vi "PDF Standard Kopf IAGnG.vi"(4 "Zeitstempel":timestamp, 5 "Gaschflasche Cluster":T2, 6 "Oprtionen Cluster":T5, 7 "Gas Komponente":cluster{"Komponente:":T4, "Konzentration":dbl} {"Konzentration" format="%#.6f"}, 8 "error in (no error)":errorcluster caption="Fehler (Eingang, kein Fehler)", 9 "LIN Pototokoll-Cluster (opotional)":T6 {"zusätzliche Zeitdauer Erster Punkt" format="%#_5g"; "Lin Modus" items=["Cal Gas to PNS", "Cal Gas to Samplepoint", "Measure"]; "Gas Ablaufdatum" format="%<%d.%m.%Y>T"; "HovaCAL Flow AutoLin"."HovaCAL Flow Input Cluster" format="%.2f"; "Gasflasche" items=["----"=10000, "IAG MG"=0, "IAG NH3 3000"=1, "IAG NH3 2000"=2, "IAG NH3 200"=3]; "Conditions:" items=["field", "laboratory"]; "Kalibrierauswahl" items=["Inaktiv", "Aktiv"]; "Anzahl Stufen" format="%#_5g"; "Zeitdauer Stufe" format="%#_5g"; "Verdünnungsgas" items=["N2", "O2"]; "Komponentenauswahl"."Konzentration" format="%#.6f"; "Gasnummer:" min=1 max=5; "Prüfgas Konzentration" format="%#.6f"; "Polynomkoeff." format="%#_18f"}, 10 "Analysator":string, 11 "Bearbeiter/in":string) -> (0 "error out":errorcluster caption="Fehler (Ausgang)", 1 "Size Cluster":T1={"Header Size"=0, "Column Ratio left"=[40.0, 60.0]}, 2 "Header Values":T3[](array[typedef]), 3 "Header Labels":string[](array[string]))   [LabVIEW 2020, in "Linearisierung v2.lvlib" / "Protokoll.lvlib"]
uses:
  Protokoll.lvlib
  Lin-Polynom Daten.ctl
  KomponentenArray.ctl
  Visualisierungs Elemente/Auswahlfeld.ctl
  Visualisierungs Elemente/Zahlen-Eingabefeld.ctl
  EPA Optionsfeld.ctl
  Gasteiler/HovaCal/AutoLin Hovacal.ctl
  Kalibrieroption.ctl
  EPA1065-307/Condition.ctl
  Seiten/System Einstellungen V2/Konfig Gasflasche.ctl
  Seiten/System Einstellungen V2/Gasflasche Auswahl.ctl
  Gasteiler/HovaCAL_Interface/Controls/Flow Einstellung.ctl
  Gasteiler/HovaCAL_Interface/Controls/Pump state.ctl
  Seiten/CalGas Aufschaltung/Lin Modus.ctl
  PDF_Interface/PDF Protokoll Standard Kopf Optionen.ctl
  Visualisierungs Elemente/String - Ausgabefeld.ctl
  PDF_Interface/PDF Protokoll Standard Kopf Gasflasche Auswahl.ctl
  Gasteiler/Aktionen FGV Gasteiler Daten.ctl
  Seiten/FT-IR/FGV FT-IR Gasliste Aktionen.ctl
  Seiten/FT-IR/FGV FT-IR Aktionen.ctl
  Gasteiler/Gasteiler.lvlib
  Seiten/FT-IR/FT-IR.lvlib
  PDF_Interface/PDF Interface.lvlib
  Linearisierung v2.lvlib
  Gasteiler/HovaCal/HovaCal.lvlib
  EPA1065-307/Linearity verification 1065-307.lvlib
  Seiten/System Einstellungen V2/System Einstellungen V2.lvlib
  Gasteiler/HovaCAL_Interface/Controls/Controls.lvlib
  Seiten/CalGas Aufschaltung/CalGas Aufschaltung.lvlib
panel:
  # "%"
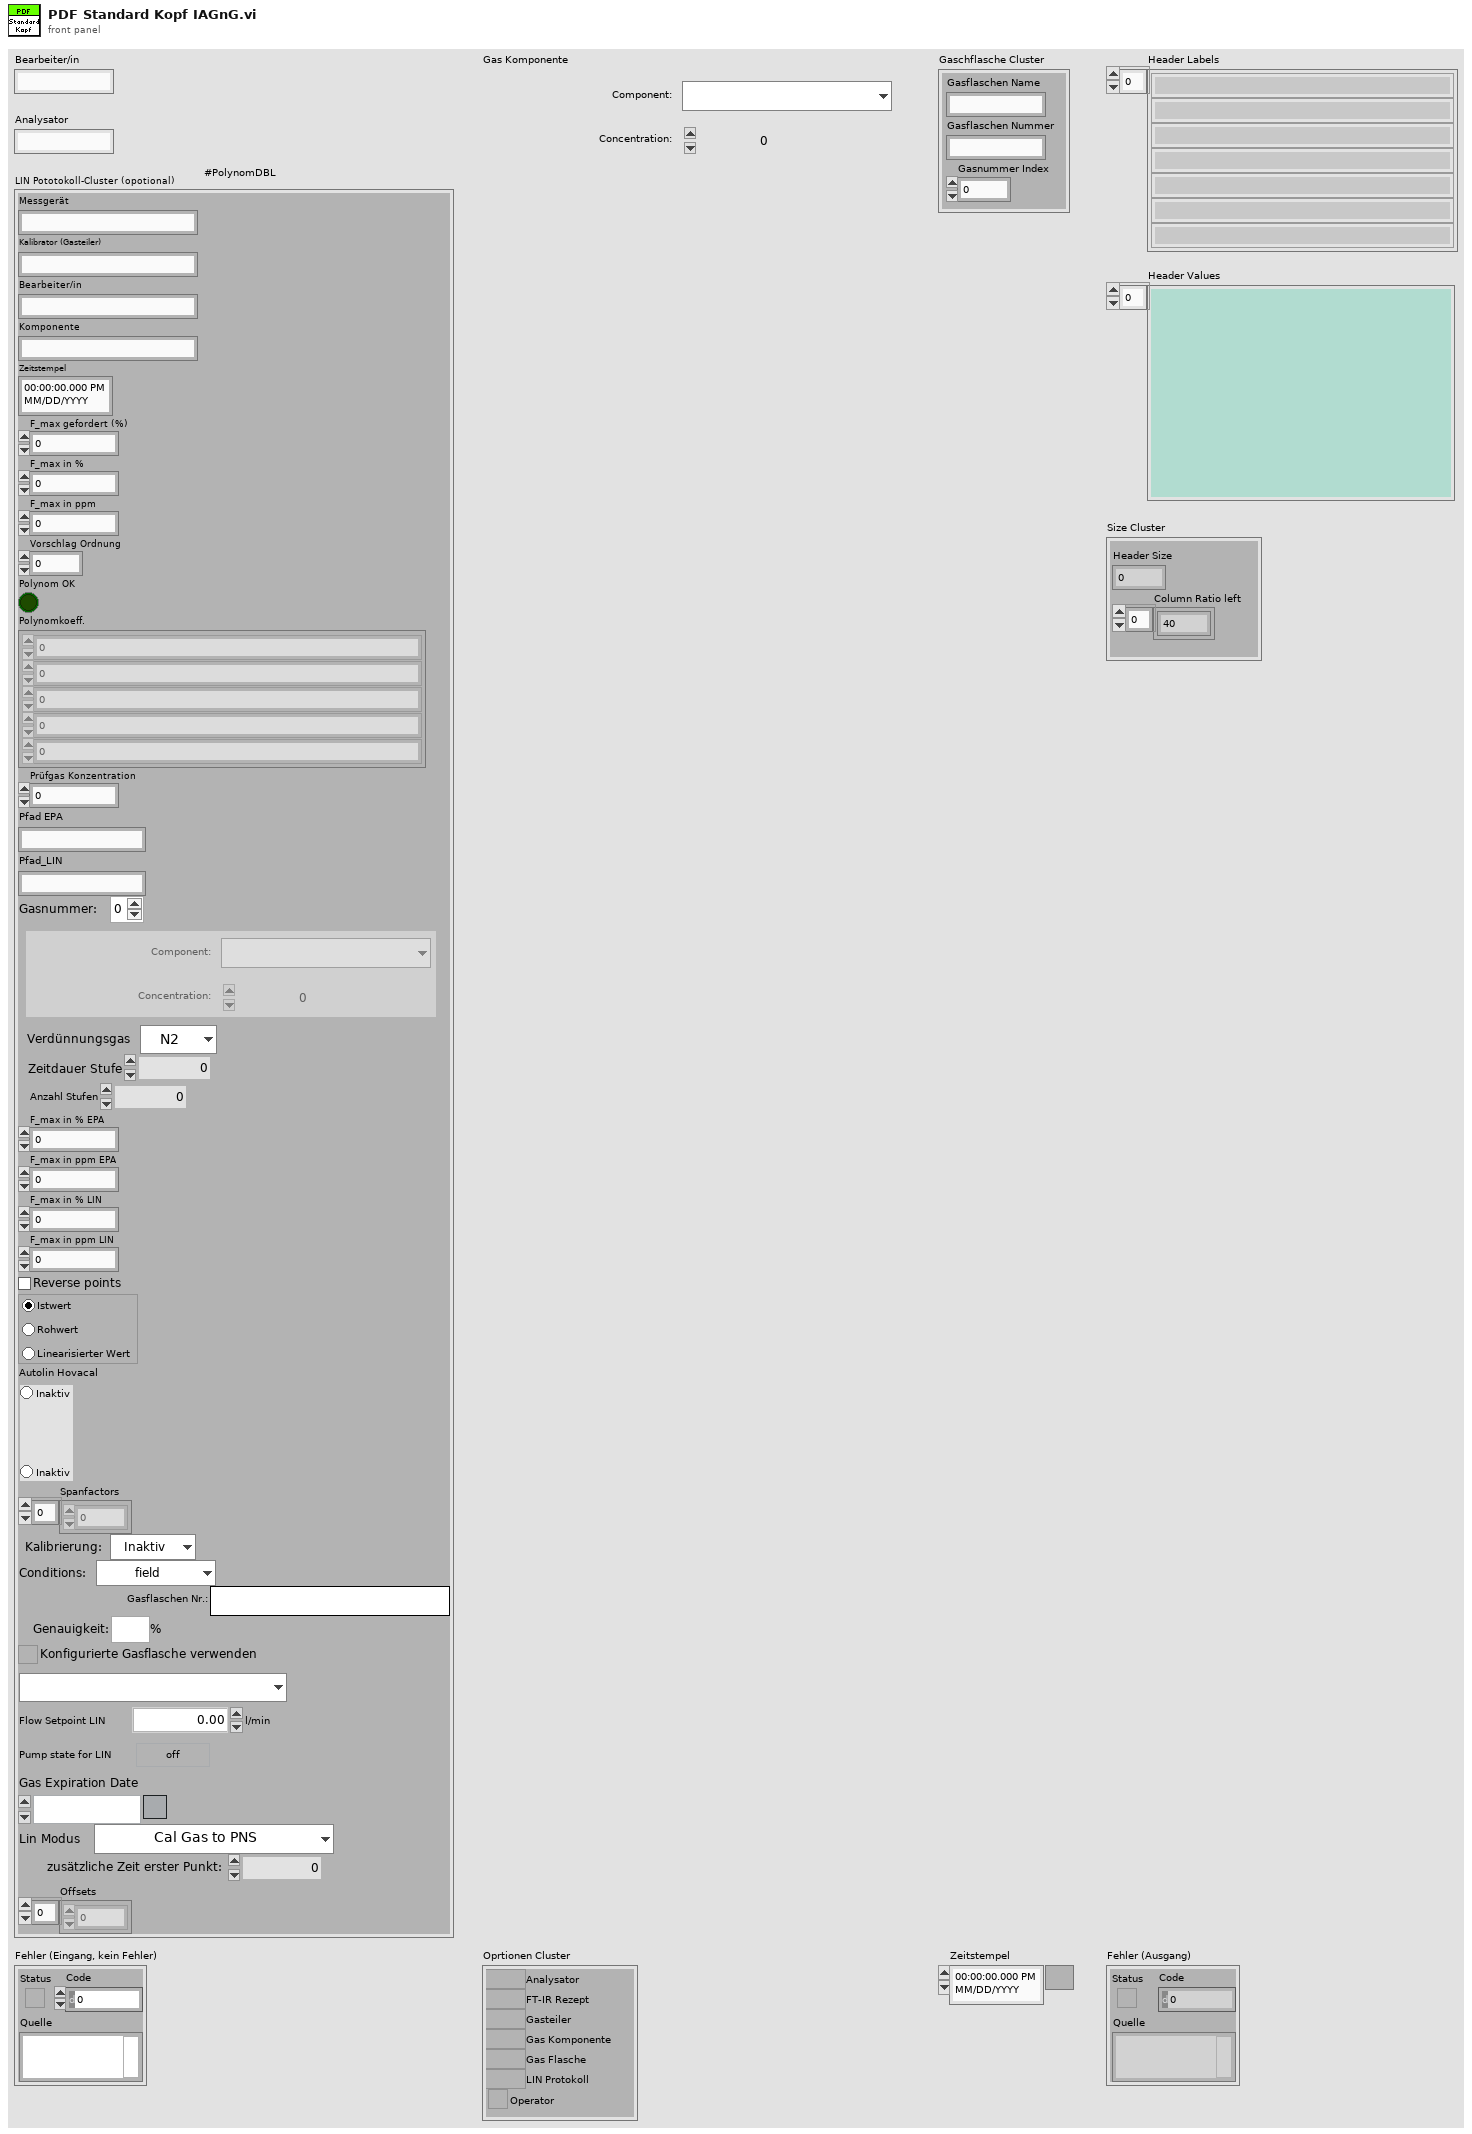
[diagram p1: front panel]
types:
  T1 = cluster{"Header Size":i32, "Column Ratio left":sgl[]}
  T2 = typedef "PDF Interface.lvlib/PDF Protokoll Standard Kopf Gasflasche Auswahl.ctl" = cluster{"Gasflaschen Name":string, "Gasflaschen Nummer":string, "Gasnummer Index":i32}
  T3 = typedef "String - Ausgabefeld.ctl" = string
  T4 = typedef "Auswahlfeld.ctl" = u16
  T5 = typedef "PDF Interface.lvlib/PDF Protokoll Standard Kopf Optionen.ctl" = cluster{"Analysator":bool, "FT-IR Rezept":bool, "Gasteiler":bool, "Gas Komponente":bool, "Gas Flasche":bool, "LIN Protokoll":bool, "Operator":bool}
  T6 = typedef "Linearisierung v2.lvlib/Lin-Polynom Daten.ctl" = cluster{"Messgerät":string, "Kalibrator (Gasteiler)":string, "Bearbeiter/in":string, "Komponente":string, "Zeitstempel":timestamp, "F_max gefordert (%)":sgl, "F_max in %":sgl, "F_max in ppm":sgl, "Vorschlag Ordnung":i32, "Polynom OK":bool, "Polynomkoeff.":dbl[], "Prüfgas Konzentration":dbl, "Pfad EPA":string, "Pfad_LIN":string, "Gasnummer:":u8, "Komponentenauswahl":T7, "Verdünnungsgas":T8, "Zeitdauer Stufe":T9, "Anzahl Stufen":T9, "F_max in % EPA":sgl, "F_max in ppm EPA":sgl, "F_max in % LIN":sgl, "F_max in ppm LIN":sgl, "Punkte umkehren":bool, "EPA Optionsfeld":T10, "Autolin Hovacal":T11, "Spanfactors":sgl[], "Kalibrierauswahl":T12, "Conditions:":T13, "Gasflaschen Nr.:":string, "Bottle Accuracy":dbl, "Konfig Gasflasche":T14, "Gasflasche":T15, "HovaCAL Flow AutoLin":T16, "MFC Output":T17, "Gas Ablaufdatum":timestamp, "Lin Modus":T18, "zusätzliche Zeitdauer Erster Punkt":sgl, "Offsets":sgl[]}
  T7 = typedef "Linearisierung v2.lvlib/KomponentenArray.ctl" = cluster{"Komponente:":T4, "Konzentration":dbl}[]
  T8 = typedef "Linearisierung v2.lvlib/Gasteiler.lvlib/Prüfgas in.ctl" = u16
  T9 = typedef "Zahlen-Eingabefeld.ctl" = sgl
  T10 = typedef "Linearisierung v2.lvlib/EPA Optionsfeld.ctl" = enum32{"Istwert", "Rohwert", "Linearisierter Wert"}
  T11 = typedef "Linearisierung v2.lvlib/Gasteiler.lvlib/HovaCal.lvlib/AutoLin Hovacal.ctl" = enum32{"Keine Auswahl", "Optionsauswahl 1", "Optionsauswahl 2"}
  T12 = typedef "Linearisierung v2.lvlib/Kalibrieroption.ctl" = u16
  T13 = typedef "Linearisierung v2.lvlib/Linearity verification 1065-307.lvlib/Condition.ctl" = u16
  T14 = typedef "System Einstellungen V2.lvlib/Konfig Gasflasche.ctl" = bool
  T15 = typedef "System Einstellungen V2.lvlib/Gasflasche Auswahl.ctl" = u16
  T16 = typedef "Linearisierung v2.lvlib/Gasteiler.lvlib/HovaCAL_Interface.lvlib/Controls.lvlib/Flow Einstellung.ctl" = cluster{"HovaCAL Flow Input Cluster":dbl}
  T17 = typedef "Linearisierung v2.lvlib/Gasteiler.lvlib/HovaCAL_Interface.lvlib/Controls.lvlib/Pump state.ctl" = cluster{"Run":bool}
  T18 = typedef "CalGas Aufschaltung.lvlib/Lin Modus.ctl" = u16
  T19 = typedef "FT-IR.lvlib/FGV FT-IR Aktionen.ctl" = enum16{"lesen", "NOG setzen", "NOS setzen", "Initialisieren", "speichern", "ALLES setzen", "FT-IR Spektrum loggen", "Komm Stoppen", "Spektrum LogKonfig"}
  T20 = typedef "FT-IR.lvlib/FGV FT-IR Gasliste Aktionen.ctl" = enum16{"lesen", "Gasliste FT-IR", "Gasliste ausgelesen", "laden", "speichern", "löschen"}
  T21 = typedef "Linearisierung v2.lvlib/Gasteiler.lvlib/Aktionen FGV Gasteiler Daten.ctl" = enum16{"lesen", "Gasteiler Daten", "Seriellen Param.", "MB-Endwert", "laden", "speichern", "Anforderung", "TCP", "Aufzeichnung Start"}
  T22 = typedef "Linearisierung v2.lvlib/Gasteiler.lvlib/Gasteiler Daten.ctl" = cluster{"Gasteiler":T23, "Gasteiler Stufen":T24, "Gasteiler Type":T25, "Konfig Gasteiler":T26, "Gasteiler Span Eingänge":u16}
  T23 = typedef "String - Eingabefeld.ctl" = string
  T24 = typedef "Linearisierung v2.lvlib/Gasteiler.lvlib/Gasteiler Stufen.ctl" = u16
  T25 = typedef "Linearisierung v2.lvlib/GasteilerType.ctl" = u16
  T26 = typedef "System Einstellungen V2.lvlib/Gasteiler Auswahl.ctl" = u16
  T27 = cluster{"Zeitstempel":timestamp, "Current Recipe":string, "Konfig Gasteiler":T26, "Aktuelle Gasliste gesamt":T3[]}
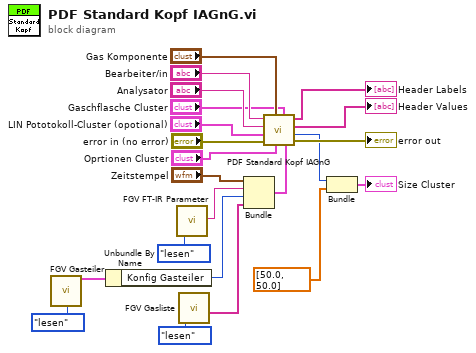
[diagram p0: block diagram]
diagram:
  n1 = call "FGV Gasteiler.vi"("Aktionen"=Aktionen_FGV_Gasteiler_Daten."lesen") -> ("Gasteiler Daten"=w21:T22)  [unwired: 11 in, 7 out]
  n2 = Unbundle By Name(w21) -> ("Konfig Gasteiler"=w14:T26)
  n3 = call "FGV FT-IR Parameter.vi"("Aktion"=FGV_FT-IR_Aktionen."lesen") -> ("Current Recipe"=w15:string)  [unwired: 11 in, 7 out]
  n4 = call "FGV Gasliste.vi"("Aktionen"=FGV_FT-IR_Gasliste_Aktionen."lesen") -> ("Aktuelle Gasliste gesamt"=w13:T3[])  [unwired: 8 in, 2 out]
  n5 = Bundle("Zeitstempel"="Zeitstempel", "Current Recipe"=w15, "Konfig Gasteiler"=w14, "Aktuelle Gasliste gesamt"=w13) -> (w12:T27)  [unwired: 1 in]
  n6 = call "PDF Standard Kopf IAGnG.vi"("L!L2 Cluster"=w12, "Gaschflasche Cluster"="Gaschflasche Cluster", "Oprtionen Cluster"="Oprtionen Cluster", "Gas Komponente"="Gas Komponente", "LIN Pototokoll-Cluster (opotional)"="LIN Pototokoll-Cluster (opotional)", "Analysator"="Analysator", "Bearbeiter/in"="Bearbeiter/in") -> ("Header Size"=w3:i32, "Header Values"=→"Header Values":T3[], "Header Labels"=→"Header Labels":string[])  [unwired: 1 in, 1 out]
  n7 = Bundle("Header Size"=w3, "Column Ratio left"=sgl[] [50.0, 50.0]) -> (→"Size Cluster":T1)  [unwired: 1 in]
  "error out" <- "error in (no error)"
